vi "MoreRecentLVVersion Test 0002.vi"(8 "error in (no error)":errorcluster) -> (0 "error out":errorcluster)   [LabVIEW 2020]
uses:
  <vilib>/addons/_JKI Toolkits/Caraya/classes/Assert/Assert.lvclass
  <vilib>/addons/_JKI Toolkits/Caraya/classes/Test/Test.lvclass
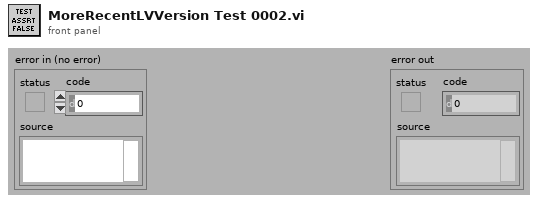
[diagram p1: front panel]
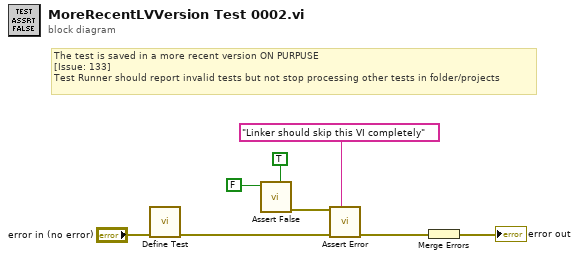
[diagram p0: block diagram]
diagram:
  # "The test is saved in a more recent version ON PURPUSE\n[Issue: 133]\nTest Runner should report invalid tests but not stop processing other tests in folder/projects"
  n1 = call <vilib>:"Define Test.vi"("error in (no error)"="error in (no error)") -> ("error out"=w1:errorcluster)  [unwired: 10 in]
  n2 = call <vilib>:"Assert False.vi"("Assert Only? (F)"=TRUE, "False?"=FALSE ("True?")) -> ("error out"=w7:errorcluster)  [unwired: 9 in]
  n3 = call <vilib>:"Assert Error.vi"("Label"="Linker should skip this VI completely", "error in (no error)"=w1, "Error?"=w7) -> ("error out"=w3:errorcluster)  [unwired: 8 in]
  n4 = Merge Errors(w3) -> (→"error out":errorcluster)
